vi "ProcessModbusUpdates.vi"(11 "MockHPILCSettings":T1={"ModbusRxDataFIFO"="MockbusPort2RxFIFO", "ModbusTxDataFIFO"="MockbusPort2TxFIFO", "BufferUpdateFIFO"="MockHPILCCommand", "Code17Memory"="MockHPILCCode17", "Code18Memory"="MockHPILCCode18", "Code65Memory"="MockHPILCCode65", "Code66Memory"="MockHPILCCode66", "Code67Memory"="MockHPILCCode67", "Code72Memory"="MockHPILCCode72", "Code80Memory"="MockHPILCCode80", "Code110Memory"="MockHPILCCode110"}) -> ()   [LabVIEW 2016, in "FPGAMockMDILC.lvlib"]
uses:
  FPGAMockMDILC.lvlib
  DataTypes/MockHPILCSettings.ctl
  <vilib>/rvi/Emulation/niFpgaSctlEmulationGetInTimedLoop.vi
  <vilib>/Utility/error.llb/Clear Errors.vi
  <vilib>/rvi/DataTransferAndStorage/Container/Common/niFpgaContainerExecOnDevCompGetState.vi
  <vilib>/rvi/Emulation/niFpgaEmulationIsFPGAContextNoSignature.vi
  <vilib>/rvi/errors/niFpgaSetErrorForExecOnDevCompSimple.vi
  <vilib>/rvi/eio/common/nirviEmuReportErrorAndStop.vi
  <vilib>/rvi/DataTransferAndStorage/Container/Common/niFpgaContainerGetUniqueNameForEmu.vi
  <vilib>/rvi/FIFO/Fifo_Resource/nirvififoEmulationSetSize.vi
  <vilib>/rvi/FIFO/Fifo_Resource/nirviFifoEmulationQueueMgr.vi
  <instcachedir>/0/nirviFifoEmulationQueueMgr_E5CAEC123FF24DC58D834DCA3CDAA9B5.lvgen/nirviFifoEmulationQueueMgr_E5CAEC123FF24DC58D834DCA3CDAA9B5_002.vi
  <vilib>/rvi/FIFO/Fifo_Resource/nirvififoEmulationDetermineInputValidOut.vi
  <vilib>/rvi/FIFO/Fifo_Resource/nirvififoEmulationCreateLock.vi
  <vilib>/rvi/Emulation/niFpgaProcessEmulError.vi
  <vilib>/rvi/FIFO/Fifo_Resource/nirvififoEmulationObtainLock.vi
  <vilib>/rvi/FIFO/Fifo_Resource/nirvififoEmulationReleaseLock.vi
  <vilib>/rvi/occurrence/nirviWaitOnOccurrenceBase.vi
  <vilib>/rvi/errors/nirviReportUnexpectedCaseInternalError.vi
  <vilib>/rvi/errors/nirviReportUnexpectedCaseInternalError (U32).vi
  <vilib>/rvi/interface/RandomDataEmulation/niFpgaRandomDataHandleErrors.vi
  <vilib>/rvi/Memory/Memory_Emulation/niFpgaMemoryEmulationCacheClearOnFirstRun.vi
  <vilib>/rvi/Memory/Memory_Emulation/nirvimemoryEmulationManagerCache_MakeExclusive.vi
  <vilib>/rvi/Memory/Memory_Emulation/niFpgaMemoryEmulationValidateCache.vi
  <vilib>/rvi/Memory/Memory_Emulation/nirvimemoryEmulationManagerCache_InsertValue.vi
  <vilib>/rvi/Memory/Memory_Emulation/nirvimemoryEmulationManagerCache_ReleaseExclusive.vi
  <vilib>/rvi/Memory/Memory_Emulation/nirvimemoryEmulationManagerCache_GetValue.vi
  <vilib>/rvi/Memory/Memory_Emulation/nirvimemoryEmulationManagerCache_SetValue.vi
  <vilib>/rvi/Emulation/niFpgaSctlEmulationResourceMgr.vi
  <vilib>/rvi/DataTransferAndStorage/Container/XNode/niFpgaContainer.xnode
  <vilib>/rvi/FIFO/Fifo_Resource/niFpgaFifoEmulationRefIn.vi
  <vilib>/rvi/Memory/Memory_Emulation/niFpgaMemoryEmulationRefIn.vi
  Common_FPGA_Modbus/FPGAModbus.lvlib
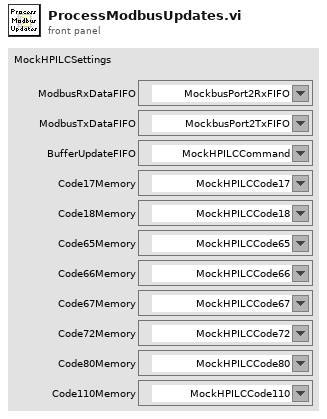
[diagram p1: front panel]
types:
  T1 = typedef "FPGAMockMDILC.lvlib/MockHPILCSettings.ctl" = cluster{"ModbusRxDataFIFO":refnum<k21>, "ModbusTxDataFIFO":refnum<k21>, "BufferUpdateFIFO":refnum<k21>, "Code17Memory":refnum<k21>, "Code18Memory":refnum<k21>, "Code65Memory":refnum<k21>, "Code66Memory":refnum<k21>, "Code67Memory":refnum<k21>, "Code72Memory":refnum<k21>, "Code80Memory":refnum<k21>, "Code110Memory":refnum<k21>}
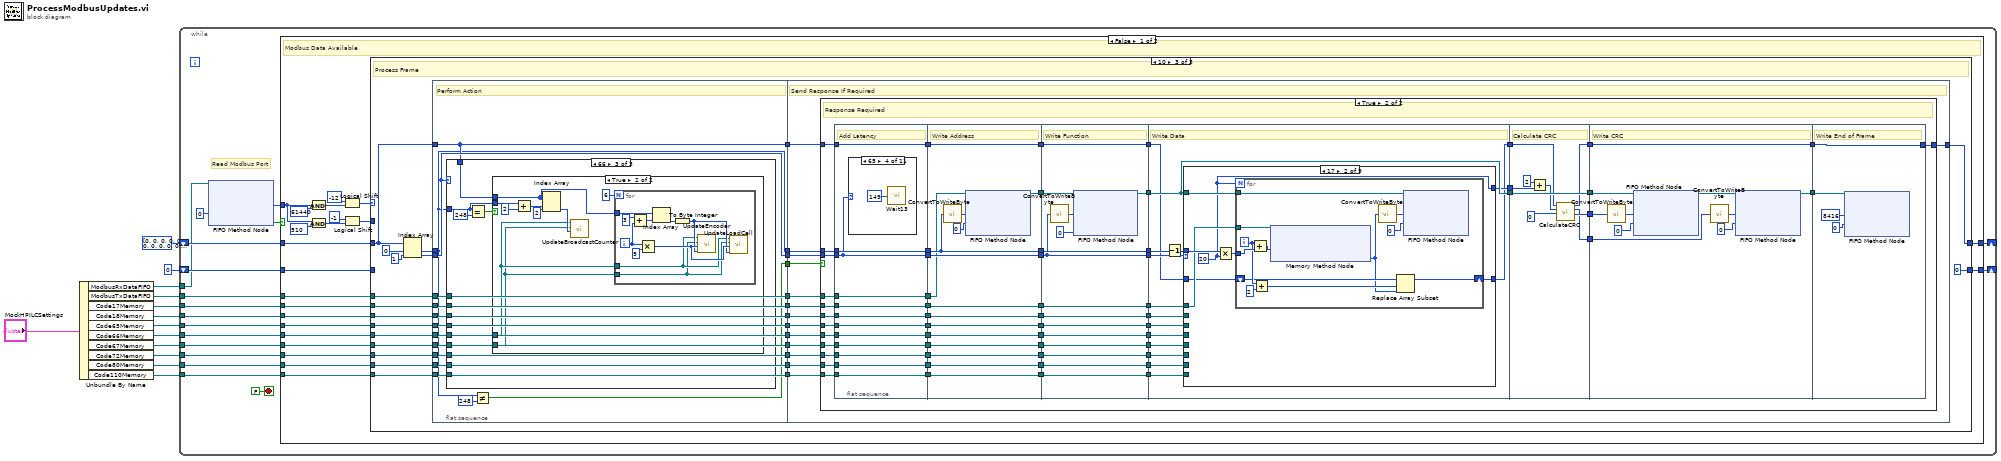
[diagram p0: block diagram]
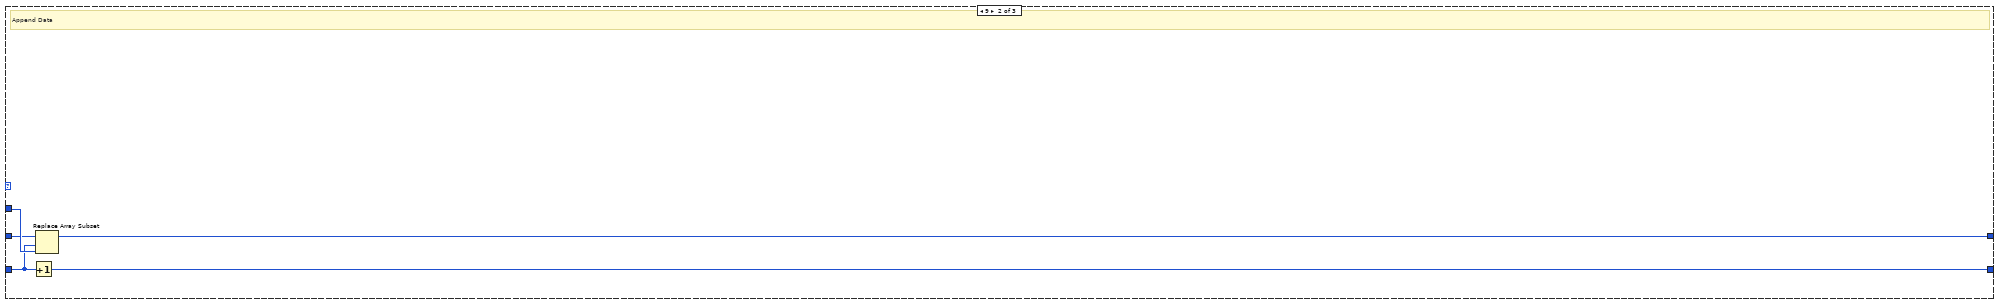
[diagram p3: hidden frame]
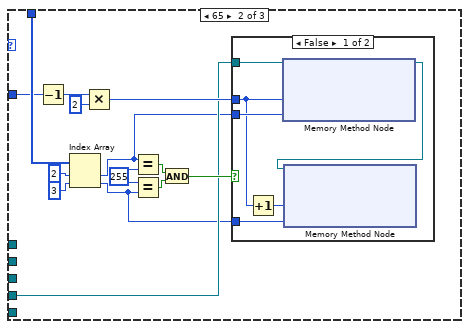
[diagram p5: hidden frame]
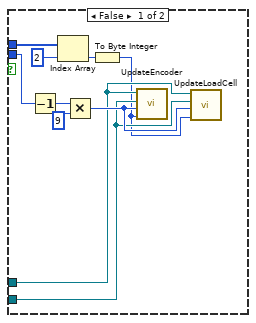
[diagram p7: hidden frame]
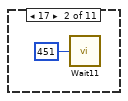
[diagram p10: hidden frame]
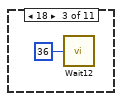
[diagram p11: hidden frame]
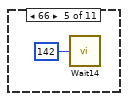
[diagram p12: hidden frame]
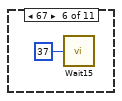
[diagram p13: hidden frame]
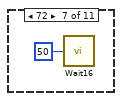
[diagram p14: hidden frame]
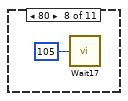
[diagram p15: hidden frame]
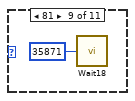
[diagram p16: hidden frame]
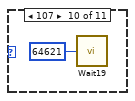
[diagram p17: hidden frame]
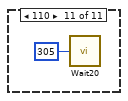
[diagram p18: hidden frame]
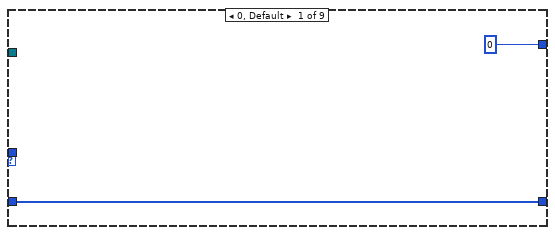
[diagram p19: hidden frame]
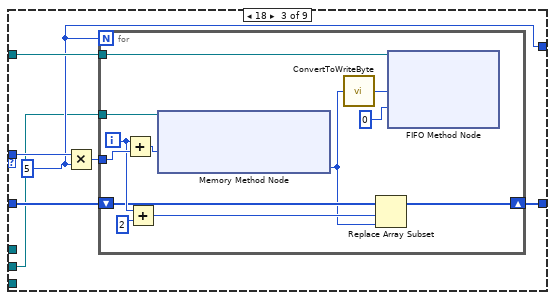
[diagram p20: hidden frame]
diagram:
  n1 = Unbundle By Name("MockHPILCSettings") -> ("ModbusRxDataFIFO"=w10:refnum<k21>, "ModbusTxDataFIFO"=w1:refnum<k21>, "Code17Memory"=w9:refnum<k21>, "Code18Memory"=w8:refnum<k21>, "Code65Memory"=w7:refnum<k21>, "Code66Memory"=w6:refnum<k21>, "Code67Memory"=w5:refnum<k21>, "Code72Memory"=w4:refnum<k21>, "Code80Memory"=w3:refnum<k21>, "Code110Memory"=w2:refnum<k21>)
  n2 = while {
    shift-right: [w26] -> _
    shift-left: u8[] [0, 0, 0, 0, 0, 0, 0, 0, 0, 0, 0, 0, 0, 0, 0, 0, 0, 0, 0, 0, 0, 0, 0, 0, 0, 0, 0, 0, 0, 0, 0, 0, 0, 0, 0, 0, 0, 0, 0, 0, 0, 0, 0, 0, 0, 0, 0, 0, 0, 0, 0, 0, 0, 0, 0, 0, 0, 0, 0, 0, 0, 0, 0, 0, 0, 0, 0, 0, 0, 0, 0, 0, 0, 0, 0, 0, 0, 0, 0, 0, 0, 0, 0, 0, 0, 0, 0, 0, 0, 0, 0, 0, 0, 0, 0, 0, 0, 0, 0, 0, 0, 0, 0, 0, 0, 0, 0, 0, 0, 0, 0, 0, 0, 0, 0, 0, 0, 0, 0, 0, 0, 0, 0, 0, 0, 0, 0, 0, 0, 0, 0, 0, 0, 0, 0, 0, 0, 0, 0, 0, 0, 0, 0, 0, 0, 0, 0, 0, 0, 0, 0, 0, 0, 0, 0, 0, 0, 0, 0, 0, 0, 0, 0, 0, 0, 0, 0, 0, 0, 0, 0, 0, 0, 0, 0, 0, 0, 0, 0, 0, 0, 0, 0, 0, 0, 0, 0, 0, 0, 0, 0, 0, 0, 0, 0, 0, 0, 0, 0, 0, 0, 0, 0, 0, 0, 0, 0, 0, 0, 0, 0, 0, 0, 0, 0, 0, 0, 0, 0, 0, 0, 0, 0, 0, 0, 0, 0, 0, 0, 0, 0, 0, 0, 0, 0, 0, 0, 0, 0, 0, 0, 0, 0, 0, 0, 0, 0, 0, 0, 0, 0, 0, 0, 0, 0, 0] -> [w27]
    shift-right: [w25] -> _
    shift-left: i16 0 -> [w28]
    tunnel: w10 -> [w23]
    tunnel: w1 -> [w22]
    tunnel: w9 -> [w21]
    tunnel: w8 -> [w20]
    tunnel: w7 -> [w19]
    tunnel: w6 -> [w18]
    tunnel: w5 -> [w17]
    tunnel: w4 -> [w16]
    tunnel: w3 -> [w15]
    tunnel: w2 -> [w14]
    stop <- FALSE stop-if-true
    # "Read Modbus Port"
    n3 = xnode ("FIFO Method Node")("Timeout"=0, "FIFO In"=w23) -> ("Element"=w29:u16, "Timed Out?"=w30:bool)  [unwired: 1 out]
    n4 = case shown="False" w30 {
      tunnel: w29 -> [w48 _]
      tunnel: w28 -> [w44 w476]
      tunnel: w27 -> [w43 w477]
      tunnel: [w42 w477] -> w26
      tunnel: [w41 w476] -> w25
      tunnel: w22 -> [w40 _]
      tunnel: w21 -> [w39 _]
      tunnel: w20 -> [w38 _]
      tunnel: w19 -> [w37 _]
      tunnel: w18 -> [w36 _]
      tunnel: w17 -> [w35 _]
      tunnel: w16 -> [w34 _]
      tunnel: w15 -> [w33 _]
      tunnel: w14 -> [w32 _]
      frame False {
        # "Modbus Data Available"
        n5 = And(x=w48, y=u16 61440) -> (x .and. y?=w52:u16)
        n6 = And(x=w48, y=u16 510) -> (x .and. y?=w47:u16)
        n7 = Logical Shift(y=i16 -12, x=w52) -> (x << y=w50:u16)
        n8 = Logical Shift(y=i16 -1, x=w47) -> (x << y=w45:u16)
        n9 = case shown="10" w50 {
          tunnel: w45 -> [_ w60 _]
          tunnel: w44 -> [w54 w57 _]
          tunnel: w43 -> [w55 w59 w75]
          tunnel: [w55 w58 w62] -> w42
          tunnel: [w54 w56 i16 0] -> w41
          tunnel: w40 -> [_ _ w84]
          tunnel: w39 -> [_ _ w83]
          tunnel: w38 -> [_ _ w82]
          tunnel: w37 -> [_ _ w81]
          tunnel: w36 -> [_ _ w80]
          tunnel: w35 -> [_ _ w79]
          tunnel: w34 -> [_ _ w78]
          tunnel: w33 -> [_ _ w77]
          tunnel: w32 -> [_ _ w76]
          frame 0, Default {
            # "Do Nothing"
          }
          frame 9 {
            # "Append Data"
            n10 = Increment(x=w57) -> (x+1=w56:i16)
            n11 = Replace Array Subset(array=w59, new element=w60, index=w57) -> (w58:u8[])
          }
          frame 10 {
            # "Process Frame"
            n12 = Index Array(array=w75, index #1=0 ("index"), index #2=1 ("index")) -> (element #1=w86:u8, element #2=w85:u8)
            n13 = flat-sequence {
              tunnel: w76 -> [w94]
              tunnel: w77 -> [w95]
              tunnel: w78 -> [w96]
              tunnel: w79 -> [w97]
              tunnel: w80 -> [w98]
              tunnel: w81 -> [w99]
              tunnel: w82 -> [w100]
              tunnel: w83 -> [w101]
              tunnel: w84 -> [w102]
              tunnel: w85 -> [w103]
              tunnel: w86 -> [w91]
              tunnel: [w91] -> w74
              tunnel: [w103] -> w73
              tunnel: [w102] -> w72
              tunnel: [w101] -> w71
              tunnel: [w100] -> w70
              tunnel: [w99] -> w69
              tunnel: [w98] -> w68
              tunnel: [w97] -> w67
              tunnel: [w96] -> w66
              tunnel: [w95] -> w65
              tunnel: [w94] -> w64
              tunnel: w75 -> [w93]
              tunnel: [w93] -> w63
              tunnel: [w90] -> w61
              tunnel: w74 -> [w171]
              tunnel: w73 -> [w170]
              tunnel: w72 -> [w169]
              tunnel: w71 -> [w168]
              tunnel: w70 -> [w167]
              tunnel: w69 -> [w166]
              tunnel: w68 -> [w165]
              tunnel: w67 -> [w164]
              tunnel: w66 -> [w163]
              tunnel: w65 -> [w162]
              tunnel: w64 -> [w161]
              tunnel: w63 -> [w172]
              tunnel: [w160] -> w62
              tunnel: w61 -> [w159]
              frame #0 {
                # "Perform Action"
                n14 = case shown="66" w103 {
                  tunnel: w91 -> [_ w105 w127]
                  tunnel: w102 -> [_ _ _]
                  tunnel: w101 -> [_ _ _]
                  tunnel: w100 -> [_ _ _]
                  tunnel: w99 -> [_ w109 _]
                  tunnel: w98 -> [_ _ w125]
                  tunnel: w97 -> [_ _ w124]
                  tunnel: w96 -> [_ _ _]
                  tunnel: w95 -> [_ _ _]
                  tunnel: w94 -> [_ _ _]
                  tunnel: w93 -> [_ w106 w126]
                  frame 0, Default {
                  }
                  frame 65 {
                    w114 = u8 255 ("y")
                    n15 = Decrement(x=w105) -> (x-1=w104:u8)
                    n16 = Index Array(array=w106, index #1=2 ("index"), index #2=3 ("index")) -> (element #1=w108:u8, element #2=w107:u8)
                    n17 = Multiply(x=w104, y=u8 2) -> (x*y=w110:u8)
                    n18 = Equal?(x=w108, y=w114) -> (x = y?=w113:bool)
                    n19 = Equal?(x=w114, y=w107) -> (x = y?=w112:bool)
                    n20 = And(x=w113, y=w112) -> (x .and. y?=w111:bool)
                    n21 = case shown="False" w111 {
                      tunnel: w110 -> [w119 _]
                      tunnel: w109 -> [w123 _]
                      tunnel: w108 -> [w122 _]
                      tunnel: w107 -> [w118 _]
                      frame False {
                        n22 = Increment(x=w119) -> (x+1=w120:u8)
                        n23 = xnode ("Memory Method Node")("Address"=w119, "Data"=w122, "Memory In"=w123) -> ("Memory Out"=w121:refnum<k21>)
                        n24 = xnode ("Memory Method Node")("Address"=w120, "Data"=w118, "Memory In"=w121) -> ()  [unwired: 1 out]
                      }
                      frame True {
                      }
                    }
                  }
                  frame 66 {
                    n25 = Equal?(x=w127, y=u8 248) -> (x = y?=w128:bool)
                    n26 = case shown="True" w128 {
                      tunnel: w126 -> [w138 w142]
                      tunnel: w125 -> [w132 w141]
                      tunnel: w124 -> [w131 w140]
                      tunnel: w127 -> [w133 w148]
                      frame False {
                        n27 = Decrement(x=w133) -> (x-1=w136:u8)
                        n28 = Index Array(array=w138, index=2) -> (element=w134:u8)
                        n29 = Multiply(x=w136, y=9) -> (x*y=w137:i32)
                        n30 = To Byte Integer(number=w134) -> (8bit integer=w130:i8)
                        n31 = call "UpdateEncoder.vi"("Steps"=w130, "Address"=w137, "Code67Memory"=w131, "Code66Memory"=w132) -> ()  [unwired: 8 in]
                        n32 = call "UpdateLoadCell.vi"("Steps"=w130, "Address"=w137, "Code67Memory"=w131, "Code66Memory"=w132) -> ()  [unwired: 8 in]
                      }
                      frame True {
                        n33 = Add(x=w148, y=u8 2) -> (x+y=w144:u8)
                        n34 = Index Array(array=w142, index #1=w144, index #2=2 ("index")) -> (element #2=w146:u8)  [unwired: 1 out]
                        n35 = call "UpdateBroadcastCounter.vi"("BroadcastCounter"=w146, "Code67Memory"=w140, "Code66Memory"=w141) -> ()  [unwired: 9 in]
                        n36 = for {
                          N: 6 -> [_]
                          tunnel: w142 -> [w156]
                          tunnel: w141 -> [w150]
                          tunnel: w140 -> [w149]
                          i -> [w153]
                          n37 = Add(x=3 ("y"), y=w153) -> (x+y=w155:i32)
                          n38 = Multiply(x=w153, y=9) -> (x*y=w158:i32)
                          n39 = Index Array(array=w156, index=w155) -> (element=w152:u8)
                          n40 = To Byte Integer(number=w152) -> (8bit integer=w151:i8)
                          n41 = call "UpdateEncoder.vi"("Steps"=w151, "Address"=w158, "Code67Memory"=w149, "Code66Memory"=w150) -> ()  [unwired: 8 in]
                          n42 = call "UpdateLoadCell.vi"("Steps"=w151, "Address"=w158, "Code67Memory"=w149, "Code66Memory"=w150) -> ()  [unwired: 8 in]
                        }
                      }
                    }
                  }
                }
                n43 = Not Equal?(x=w91, y=u8 248) -> (x != y?=w90:bool)
              }
              frame #1 {
                # "Send Response If Required"
                n44 = case shown="True" w159 {
                  tunnel: w172 -> [w173 w186]
                  tunnel: w171 -> [_ w185]
                  tunnel: w170 -> [_ w184]
                  tunnel: w169 -> [_ w183]
                  tunnel: w168 -> [_ w182]
                  tunnel: w167 -> [_ w181]
                  tunnel: w166 -> [_ w180]
                  tunnel: w165 -> [_ w179]
                  tunnel: w164 -> [_ w178]
                  tunnel: w163 -> [_ w177]
                  tunnel: w162 -> [_ w176]
                  tunnel: w161 -> [_ w175]
                  tunnel: [w173 w174] -> w160
                  frame False {
                    # "Response Not Required"
                  }
                  frame True {
                    # "Response Required"
                    n45 = flat-sequence {
                      tunnel: [w242] -> w231
                      tunnel: [w241] -> w230
                      tunnel: [w240] -> w229
                      tunnel: [w239] -> w228
                      tunnel: [w238] -> w227
                      tunnel: [w237] -> w226
                      tunnel: [w236] -> w225
                      tunnel: [w235] -> w224
                      tunnel: [w234] -> w223
                      tunnel: [w233] -> w222
                      tunnel: [w232] -> w221
                      tunnel: [w243] -> w220
                      tunnel: w186 -> [w243]
                      tunnel: w185 -> [w242]
                      tunnel: w184 -> [w241]
                      tunnel: w183 -> [w240]
                      tunnel: w182 -> [w239]
                      tunnel: w181 -> [w238]
                      tunnel: w180 -> [w237]
                      tunnel: w179 -> [w236]
                      tunnel: w178 -> [w235]
                      tunnel: w177 -> [w234]
                      tunnel: w176 -> [w233]
                      tunnel: w175 -> [w232]
                      tunnel: [w268] -> w219
                      tunnel: [w265] -> w218
                      tunnel: [w264] -> w217
                      tunnel: [w262] -> w216
                      tunnel: [w261] -> w215
                      tunnel: [w260] -> w214
                      tunnel: [w259] -> w213
                      tunnel: [w258] -> w212
                      tunnel: [w257] -> w211
                      tunnel: [w256] -> w210
                      tunnel: [w255] -> w209
                      tunnel: w231 -> [w264]
                      tunnel: w230 -> [w265]
                      tunnel: w229 -> [w263]
                      tunnel: w228 -> [w262]
                      tunnel: w227 -> [w261]
                      tunnel: w226 -> [w260]
                      tunnel: w225 -> [w259]
                      tunnel: w224 -> [w258]
                      tunnel: w223 -> [w257]
                      tunnel: w222 -> [w256]
                      tunnel: w221 -> [w255]
                      tunnel: [w254] -> w208
                      tunnel: w220 -> [w254]
                      tunnel: w219 -> [w280]
                      tunnel: w218 -> [w278]
                      tunnel: w217 -> [w283]
                      tunnel: [w279] -> w207
                      tunnel: [w278] -> w206
                      tunnel: [w283] -> w205
                      tunnel: [w277] -> w204
                      tunnel: w216 -> [w277]
                      tunnel: [w276] -> w203
                      tunnel: w215 -> [w276]
                      tunnel: [w275] -> w202
                      tunnel: w214 -> [w275]
                      tunnel: [w274] -> w201
                      tunnel: w213 -> [w274]
                      tunnel: [w273] -> w200
                      tunnel: w212 -> [w273]
                      tunnel: [w272] -> w199
                      tunnel: w211 -> [w272]
                      tunnel: [w271] -> w198
                      tunnel: w210 -> [w271]
                      tunnel: [w270] -> w197
                      tunnel: w209 -> [w270]
                      tunnel: [w269] -> w196
                      tunnel: w208 -> [w269]
                      tunnel: w207 -> [w298]
                      tunnel: w206 -> [w289]
                      tunnel: w205 -> [w287]
                      tunnel: [w298] -> w195
                      tunnel: w204 -> [w297]
                      tunnel: w203 -> [w296]
                      tunnel: w202 -> [w295]
                      tunnel: w201 -> [w294]
                      tunnel: w200 -> [w293]
                      tunnel: w199 -> [w292]
                      tunnel: w198 -> [w291]
                      tunnel: w197 -> [w290]
                      tunnel: [w288] -> w194
                      tunnel: w196 -> [w285]
                      tunnel: [w284] -> w193
                      tunnel: w195 -> [w461]
                      tunnel: [w461] -> w192
                      tunnel: [w457] -> w191
                      tunnel: [w456] -> w190
                      tunnel: w194 -> [w458]
                      tunnel: [w453] -> w189
                      tunnel: w193 -> [w454]
                      tunnel: w192 -> [w466]
                      tunnel: w191 -> [w465]
                      tunnel: w190 -> [w464]
                      tunnel: [w463] -> w188
                      tunnel: w189 -> [w462]
                      tunnel: [w462] -> w187
                      tunnel: w188 -> [w475]
                      tunnel: [w472] -> _
                      tunnel: w187 -> [w472]
                      tunnel: [w472] -> w174
                      frame #0 {
                        # "Add Latency"
                        n46 = case shown="65" w241 {
                          frame 0, Default {
                          }
                          frame 17 {
                            n47 = call "Wait11"("Count(uSec)"=u32 451) -> ()  [unwired: 1 out]
                          }
                          frame 18 {
                            n48 = call "Wait12"("Count(uSec)"=u32 36) -> ()  [unwired: 1 out]
                          }
                          frame 65 {
                            n49 = call "Wait13"("Count(uSec)"=u32 149) -> ()  [unwired: 1 out]
                          }
                          frame 66 {
                            n50 = call "Wait14"("Count(uSec)"=u32 142) -> ()  [unwired: 1 out]
                          }
                          frame 67 {
                            n51 = call "Wait15"("Count(uSec)"=u32 37) -> ()  [unwired: 1 out]
                          }
                          frame 72 {
                            n52 = call "Wait16"("Count(uSec)"=u32 50) -> ()  [unwired: 1 out]
                          }
                          frame 80 {
                            n53 = call "Wait17"("Count(uSec)"=u32 105) -> ()  [unwired: 1 out]
                          }
                          frame 81 {
                            n54 = call "Wait18"("Count(uSec)"=u32 35871) -> ()  [unwired: 1 out]
                          }
                          frame 107 {
                            n55 = call "Wait19"("Count(uSec)"=u32 64621) -> ()  [unwired: 1 out]
                          }
                          frame 110 {
                            n56 = call "Wait20"("Count(uSec)"=u32 305) -> ()  [unwired: 1 out]
                          }
                        }
                      }
                      frame #1 {
                        # "Write Address"
                        n57 = call "ConvertToWriteByte.vi"("Input"=w264) -> ("Output"=w267:u16)
                        n58 = xnode ("FIFO Method Node")("Element"=w267, "Timeout"=0, "FIFO In"=w263) -> ("FIFO Out"=w268:refnum<k21>)  [unwired: 1 out]
                      }
                      frame #2 {
                        # "Write Function"
                        n59 = call "ConvertToWriteByte.vi"("Input"=w278) -> ("Output"=w281:u16)
                        n60 = xnode ("FIFO Method Node")("Element"=w281, "Timeout"=0, "FIFO In"=w280) -> ("FIFO Out"=w279:refnum<k21>)  [unwired: 1 out]
                      }
                      frame #3 {
                        # "Write Data"
                        n61 = Decrement(x=w287) -> (x-1=w286:u8)
                        n62 = case shown="17" w289 {
                          tunnel: w286 -> [_ w306 w325 w339 w363 w382 w401 w420 w439]
                          tunnel: w298 -> [_ w305 w324 w344 w362 w381 w400 w419 w438]
                          tunnel: w297 -> [_ w304 _ _ _ _ _ _ _]
                          tunnel: w296 -> [_ _ w320 _ _ _ _ _ _]
                          tunnel: w295 -> [_ _ _ w340 _ _ _ _ _]
                          tunnel: w294 -> [_ _ _ _ w358 _ _ _ _]
                          tunnel: w293 -> [_ _ _ _ _ w377 _ _ _]
                          tunnel: w292 -> [_ _ _ _ _ _ w396 _ _]
                          tunnel: w291 -> [_ _ _ _ _ _ _ w415 _]
                          tunnel: w290 -> [_ _ _ _ _ _ _ _ w434]
                          tunnel: [u8 0 ("y") w303 w323 w343 w361 w380 w399 w418 w437] -> w288
                          tunnel: w285 -> [w299 w302 w322 w342 w360 w379 w398 w417 w436]
                          tunnel: [w299 w301 w321 w341 w359 w378 w397 w416 w435] -> w284
                          frame 0, Default {
                          }
                          frame 17 {
                            w303 = u8 20 ("y")
                            n63 = Multiply(x=w306, y=w303) -> (x*y=w307:u8)
                            n64 = for {
                              N: w303 -> [_]
                              tunnel: w307 -> [w318]
                              tunnel: w305 -> [w316]
                              tunnel: w304 -> [w314]
                              shift-right: [w308] -> w301
                              shift-left: w302 -> [w311]
                              i -> [w313]
                              n65 = Add(x=w313, y=w318) -> (x+y=w319:i32)
                              n66 = Add(x=w313, y=2) -> (x+y=w310:i32)
                              n67 = xnode ("Memory Method Node")("Address"=w319, "Memory In"=w314) -> ("Data"=w309:u8)  [unwired: 1 out]
                              n68 = call "ConvertToWriteByte.vi"("Input"=w309) -> ("Output"=w317:u16)
                              n69 = Replace Array Subset(array=w311, new element=w309, index=w310) -> (w308:u8[])
                              n70 = xnode ("FIFO Method Node")("Element"=w317, "Timeout"=0, "FIFO In"=w316) -> ()  [unwired: 2 out]
                            }
                          }
                          frame 18 {
                            w323 = u8 5 ("y")
                            n71 = Multiply(x=w325, y=w323) -> (x*y=w326:u8)
                            n72 = for {
                              N: w323 -> [_]
                              tunnel: w326 -> [w337]
                              tunnel: w324 -> [w335]
                              tunnel: w320 -> [w333]
                              shift-right: [w327] -> w321
                              shift-left: w322 -> [w330]
                              i -> [w332]
                              n73 = Add(x=w332, y=w337) -> (x+y=w338:i32)
                              n74 = Add(x=w332, y=2) -> (x+y=w329:i32)
                              n75 = xnode ("Memory Method Node")("Address"=w338, "Memory In"=w333) -> ("Data"=w328:u8)  [unwired: 1 out]
                              n76 = call "ConvertToWriteByte.vi"("Input"=w328) -> ("Output"=w336:u16)
                              n77 = Replace Array Subset(array=w330, new element=w328, index=w329) -> (w327:u8[])
                              n78 = xnode ("FIFO Method Node")("Element"=w336, "Timeout"=0, "FIFO In"=w335) -> ()  [unwired: 2 out]
                            }
                          }
                          frame 65 {
                            w343 = u8 2 ("y")
                            n79 = Multiply(x=w339, y=w343) -> (x*y=w345:u8)
                            n80 = for {
                              N: w343 -> [_]
                              tunnel: w345 -> [w356]
                              tunnel: w344 -> [w354]
                              tunnel: w340 -> [w352]
                              shift-right: [w346] -> w341
                              shift-left: w342 -> [w349]
                              i -> [w351]
                              n81 = Add(x=w351, y=w356) -> (x+y=w357:i32)
                              n82 = Add(x=w351, y=2) -> (x+y=w348:i32)
                              n83 = xnode ("Memory Method Node")("Address"=w357, "Memory In"=w352) -> ("Data"=w347:u8)  [unwired: 1 out]
                              n84 = call "ConvertToWriteByte.vi"("Input"=w347) -> ("Output"=w355:u16)
                              n85 = Replace Array Subset(array=w349, new element=w347, index=w348) -> (w346:u8[])
                              n86 = xnode ("FIFO Method Node")("Element"=w355, "Timeout"=0, "FIFO In"=w354) -> ()  [unwired: 2 out]
                            }
                          }
                          frame 66 {
                            w361 = u8 9 ("y")
                            n87 = Multiply(x=w363, y=w361) -> (x*y=w364:u8)
                            n88 = for {
                              N: w361 -> [_]
                              tunnel: w364 -> [w375]
                              tunnel: w362 -> [w373]
                              tunnel: w358 -> [w371]
                              shift-right: [w365] -> w359
                              shift-left: w360 -> [w368]
                              i -> [w370]
                              n89 = Add(x=w370, y=w375) -> (x+y=w376:i32)
                              n90 = Add(x=w370, y=2) -> (x+y=w367:i32)
                              n91 = xnode ("Memory Method Node")("Address"=w376, "Memory In"=w371) -> ("Data"=w366:u8)  [unwired: 1 out]
                              n92 = call "ConvertToWriteByte.vi"("Input"=w366) -> ("Output"=w374:u16)
                              n93 = Replace Array Subset(array=w368, new element=w366, index=w367) -> (w365:u8[])
                              n94 = xnode ("FIFO Method Node")("Element"=w374, "Timeout"=0, "FIFO In"=w373) -> ()  [unwired: 2 out]
                            }
                          }
                          frame 67 {
                            w380 = u8 9 ("y")
                            n95 = Multiply(x=w382, y=w380) -> (x*y=w383:u8)
                            n96 = for {
                              N: w380 -> [_]
                              tunnel: w383 -> [w394]
                              tunnel: w381 -> [w392]
                              tunnel: w377 -> [w390]
                              shift-right: [w384] -> w378
                              shift-left: w379 -> [w387]
                              i -> [w389]
                              n97 = Add(x=w389, y=w394) -> (x+y=w395:i32)
                              n98 = Add(x=w389, y=2) -> (x+y=w386:i32)
                              n99 = xnode ("Memory Method Node")("Address"=w395, "Memory In"=w390) -> ("Data"=w385:u8)  [unwired: 1 out]
                              n100 = call "ConvertToWriteByte.vi"("Input"=w385) -> ("Output"=w393:u16)
                              n101 = Replace Array Subset(array=w387, new element=w385, index=w386) -> (w384:u8[])
                              n102 = xnode ("FIFO Method Node")("Element"=w393, "Timeout"=0, "FIFO In"=w392) -> ()  [unwired: 2 out]
                            }
                          }
                          frame 72 {
                            w399 = u8 1 ("y")
                            n103 = Multiply(x=w401, y=w399) -> (x*y=w402:u8)
                            n104 = for {
                              N: w399 -> [_]
                              tunnel: w402 -> [w413]
                              tunnel: w400 -> [w411]
                              tunnel: w396 -> [w409]
                              shift-right: [w403] -> w397
                              shift-left: w398 -> [w406]
                              i -> [w408]
                              n105 = Add(x=w408, y=w413) -> (x+y=w414:i32)
                              n106 = Add(x=w408, y=2) -> (x+y=w405:i32)
                              n107 = xnode ("Memory Method Node")("Address"=w414, "Memory In"=w409) -> ("Data"=w404:u8)  [unwired: 1 out]
                              n108 = call "ConvertToWriteByte.vi"("Input"=w404) -> ("Output"=w412:u16)
                              n109 = Replace Array Subset(array=w406, new element=w404, index=w405) -> (w403:u8[])
                              n110 = xnode ("FIFO Method Node")("Element"=w412, "Timeout"=0, "FIFO In"=w411) -> ()  [unwired: 2 out]
                            }
                          }
                          frame 80 {
                            w418 = u8 1 ("y")
                            n111 = Multiply(x=w420, y=w418) -> (x*y=w421:u8)
                            n112 = for {
                              N: w418 -> [_]
                              tunnel: w421 -> [w432]
                              tunnel: w419 -> [w430]
                              tunnel: w415 -> [w428]
                              shift-right: [w422] -> w416
                              shift-left: w417 -> [w425]
                              i -> [w427]
                              n113 = Add(x=w427, y=w432) -> (x+y=w433:i32)
                              n114 = Add(x=w427, y=2) -> (x+y=w424:i32)
                              n115 = xnode ("Memory Method Node")("Address"=w433, "Memory In"=w428) -> ("Data"=w423:u8)  [unwired: 1 out]
                              n116 = call "ConvertToWriteByte.vi"("Input"=w423) -> ("Output"=w431:u16)
                              n117 = Replace Array Subset(array=w425, new element=w423, index=w424) -> (w422:u8[])
                              n118 = xnode ("FIFO Method Node")("Element"=w431, "Timeout"=0, "FIFO In"=w430) -> ()  [unwired: 2 out]
                            }
                          }
                          frame 110 {
                            w437 = u8 96 ("y")
                            n119 = Multiply(x=w439, y=w437) -> (x*y=w440:u8)
                            n120 = for {
                              N: w437 -> [_]
                              tunnel: w440 -> [w451]
                              tunnel: w438 -> [w449]
                              tunnel: w434 -> [w447]
                              shift-right: [w441] -> w435
                              shift-left: w436 -> [w444]
                              i -> [w446]
                              n121 = Add(x=w446, y=w451) -> (x+y=w452:i32)
                              n122 = Add(x=w446, y=2) -> (x+y=w443:i32)
                              n123 = xnode ("Memory Method Node")("Address"=w452, "Memory In"=w447) -> ("Data"=w442:u8)  [unwired: 1 out]
                              n124 = call "ConvertToWriteByte.vi"("Input"=w442) -> ("Output"=w450:u16)
                              n125 = Replace Array Subset(array=w444, new element=w442, index=w443) -> (w441:u8[])
                              n126 = xnode ("FIFO Method Node")("Element"=w450, "Timeout"=0, "FIFO In"=w449) -> ()  [unwired: 2 out]
                            }
                          }
                        }
                      }
                      frame #4 {
                        # "Calculate CRC"
                        n127 = Add(x=i16 2, y=w458) -> (x+y=w455:i16)
                        n128 = call "CalculateCRC.vi"("StartIndex"=0, "Length"=w455, "Data"=w454) -> ("LSB"=w457:u8, "MSB"=w456:u8, "Data Out"=w453:u8[])  [unwired: 6 in]
                      }
                      frame #5 {
                        # "Write CRC"
                        n129 = call "ConvertToWriteByte.vi"("Input"=w465) -> ("Output"=w467:u16)
                        n130 = xnode ("FIFO Method Node")("Element"=w467, "Timeout"=0, "FIFO In"=w466) -> ("FIFO Out"=w469:refnum<k21>)  [unwired: 1 out]
                        n131 = call "ConvertToWriteByte.vi"("Input"=w464) -> ("Output"=w468:u16)
                        n132 = xnode ("FIFO Method Node")("Element"=w468, "Timeout"=0, "FIFO In"=w469) -> ("FIFO Out"=w463:refnum<k21>)  [unwired: 1 out]
                      }
                      frame #6 {
                        # "Write End of Frame"
                        n133 = xnode ("FIFO Method Node")("Element"=u16 8416, "Timeout"=0, "FIFO In"=w475) -> ()  [unwired: 2 out]
                      }
                    }
                  }
                }
              }
            }
          }
        }
      }
      frame True {
        # "Modbus Data Not Available"
      }
    }
  }
